vi "Main.vi"() -> ()   [LabVIEW 2017]
uses:
  Experiment States.ctl
  <vilib>/DAQmx/read.llb/DAQmx Read (Analog 1D DBL NChan 1Samp).vi
  <vilib>/DAQmx/miscellaneous.llb/DAQmx Fill In Error Info.vi
panel:
  in  "Lower Tower Delta P Channel":tag="cDAQ1Mod1/ai8"
  in  "Upper Tower Delta P Channel":tag="cDAQ1Mod1/ai8"
  out "Lower Tower Delta P":dbl(knob) scale=0.0..10.0
  out "Upper Tower Delta P":dbl(knob) scale=0.0..10.0
  in  "Maximum CO2 Concentration":dbl=20.0
  out "CO2 Concentration":cluster{"X":dbl, "Y":dbl}[](graph)
  in  "IR Sensor Channel":tag="cDAQ1Mod1/ai8"
  in  "End Experiment?":bool
  in  "Start":bool
  # "Set the above values before \nstarting the experiment"
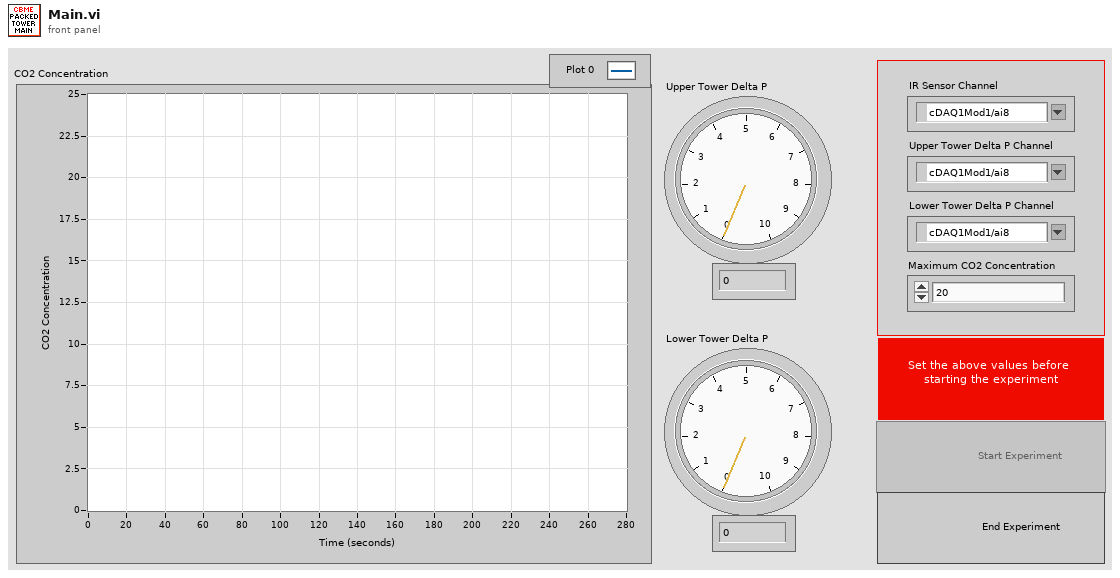
[diagram p1: front panel]
types:
  T1 = typedef "Experiment States.ctl" = enum16{"Setup", "Data Collection", "Export", "Finish"}
  T2 = enum8{"Enabled", "Disabled", "Disabled and Grayed Out"}
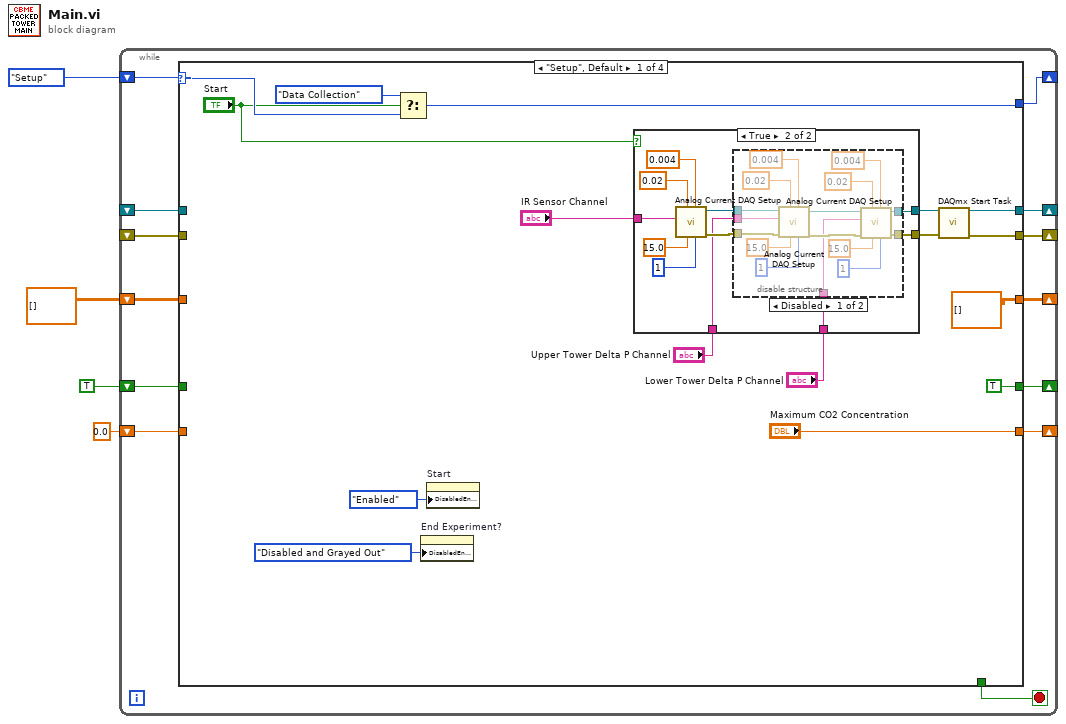
[diagram p0: block diagram]
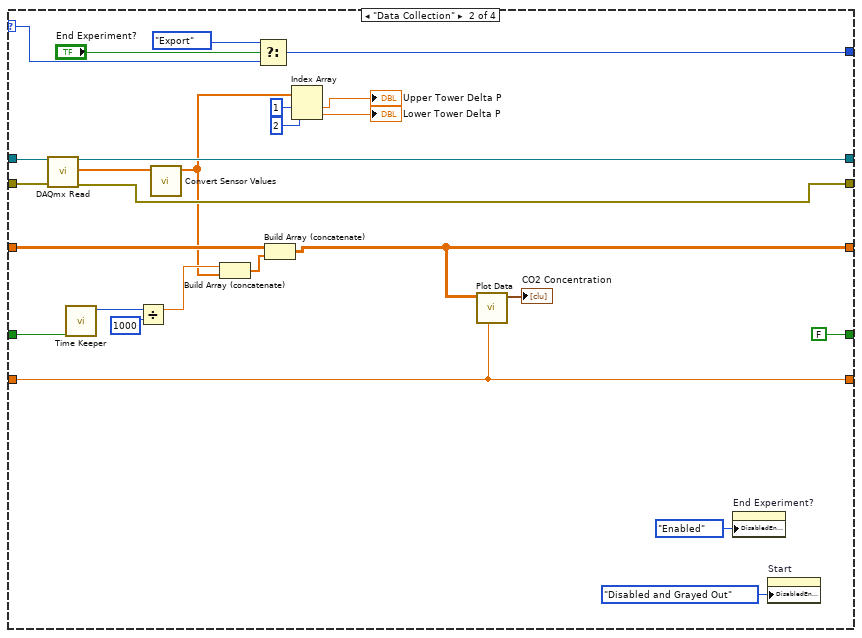
[diagram p4: hidden frame]
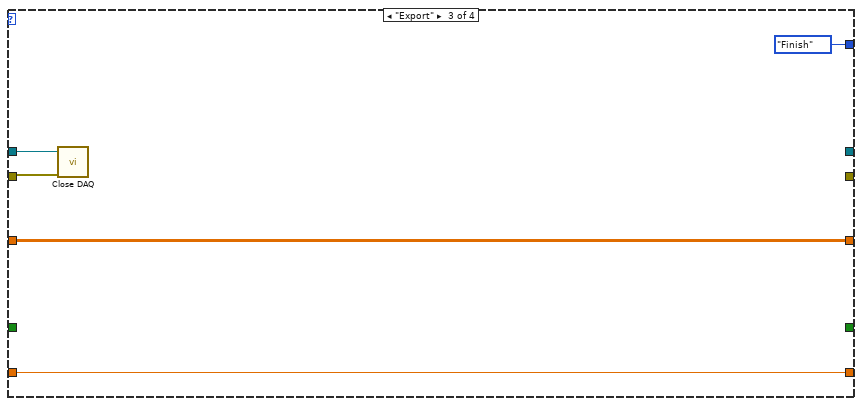
[diagram p5: hidden frame]
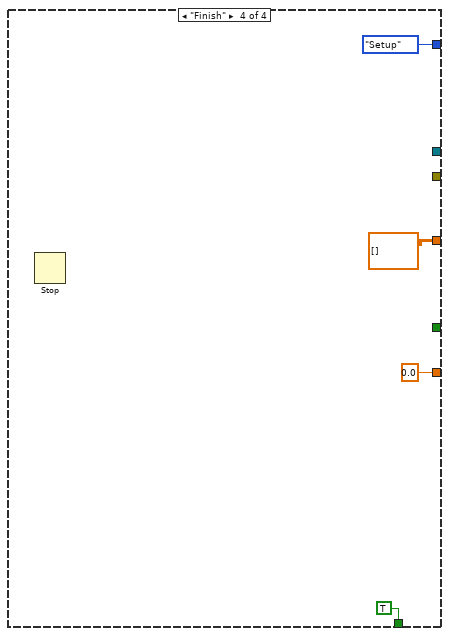
[diagram p6: hidden frame]
diagram:
  n1 = while {
    shift-right: [w16] -> _
    shift-left: Experiment_States."Setup" ("Enum") -> [w17]
    shift-right: [w13] -> _
    shift-left: _ -> [w11]
    shift-right: [w14] -> _
    shift-left: _ -> [w12]
    shift-right: [w5] -> _
    shift-left: TRUE ("Reset?") -> [w10]
    shift-right: [w8] -> _
    shift-left: dbl[][] [] -> [w9]
    shift-right: [w7] -> _
    shift-left: 0.0 ("IR Sensor Max Value") -> [w6]
    stop <- w15 stop-if-true
    n2 = case shown="\"Setup\", Default" w17 {
      selector: w17 -> [w33 w87 _ _]
      tunnel: [w31 w85 Experiment_States."Finish" ("Enum") Experiment_States."Setup" ("Enum")] -> w16
      tunnel: [_ _ _ TRUE] -> w15
      tunnel: [w27 w81 _ _] -> w14
      tunnel: [w26 w80 _ _] -> w13
      tunnel: w12 -> [_ w83 w92 _]
      tunnel: w11 -> [_ w82 w91 _]
      tunnel: w10 -> [_ w79 _ _]
      tunnel: w9 -> [_ w77 w90 _]
      tunnel: [dbl[][] [] w69 w90 dbl[][] []] -> w8
      tunnel: ["Maximum CO2 Concentration" w74 w89 0.0 ("IR Sensor Max Value")] -> w7
      tunnel: w6 -> [_ w74 w89 _]
      tunnel: [TRUE ("Reset?") FALSE ("Reset?") _ _] -> w5
      frame "Setup", Default {
        n3 = Select(t=Experiment_States."Data Collection", s="Start", f=w33) -> (s? t:f=w31:T1)
        n4 = property on="End Experiment?" class="Bool"("DisabledEnum"=T2."Disabled and Grayed Out" ("Disabled")) -> ()  [unwired: 2 in, 2 out]
        n5 = property on="Start" class="Bool"("DisabledEnum"=T2."Enabled" ("Disabled")) -> ()  [unwired: 2 in, 2 out]
        n6 = case shown="True" "Start" {
          tunnel: [_ w36] -> w29
          tunnel: [_ w35] -> w28
          tunnel: "IR Sensor Channel" -> [_ w42]
          tunnel: "Upper Tower Delta P Channel" -> [_ w37]
          tunnel: "Lower Tower Delta P Channel" -> [_ w34]
          frame False {
          }
          frame True {
            n7 = call "Analog Current DAQ Setup.vi"("samples per channel"=1, "minimum value"=0.004, "rate"=15.0 ("Sample Rate"), "maximum value"=0.02, "physical channels"=w42) -> ("error out"=w38:errorcluster, "task out"=w39:refnum<k21>)  [unwired: 5 in]
            n8 = disable-structure shown="Disabled" {
              disable-tunnel: w39 -> [w56 w62]
              disable-tunnel: w38 -> [w55 w61]
              disable-tunnel: w37 -> [w54 _]
              disable-tunnel: [w47 w62] -> w36
              disable-tunnel: [w46 w61] -> w35
              disable-tunnel: w34 -> [w45 _]
              frame Disabled {
                n9 = call "Analog Current DAQ Setup.vi"("samples per channel"=1, "minimum value"=0.004, "rate"=15.0 ("Sample Rate"), "maximum value"=0.02, "error in"=w55, "physical channels"=w54, "task in"=w56) -> ("error out"=w48:errorcluster, "task out"=w49:refnum<k21>)  [unwired: 3 in]
                n10 = call "Analog Current DAQ Setup.vi"("samples per channel"=1, "minimum value"=0.004, "rate"=15.0 ("Sample Rate"), "maximum value"=0.02, "error in"=w48, "physical channels"=w45, "task in"=w49) -> ("error out"=w46:errorcluster, "task out"=w47:refnum<k21>)  [unwired: 3 in]
              }
              frame Enabled {
              }
            }
          }
        }
        n11 = call <vilib>:"DAQmx Start Task.vi"("task/channels in"=w29, "error in"=w28) -> ("task out"=w27:refnum<k21>, "error out"=w26:errorcluster)  [unwired: 12 in]
      }
      frame "Data Collection" {
        n12 = call-poly <vilib>:"DAQmx Read.vi"("task/channels in"=w83, "error in"=w82) -> ("task out"=w81:refnum<k21>, "data"=w64:dbl[], "error out"=w80:errorcluster)  [unwired: 11 in]
        n13 = call "Time Keeper.vi"("Reset?"=w79) -> ("Time Elapsed (ms)"=w78:u32)  [unwired: 10 in]
        n14 = Divide(x=w78, y=u32 1000) -> (x/y=w71:dbl)
        n15 = call "Convert Sensor Values.vi"("ECE Units"=w64) -> ("CBME Units"=w63:dbl[])  [unwired: 10 in]
        n16 = Build Array (concatenate)(w71, w63) -> (w76:dbl[])
        n17 = Select(t=Experiment_States."Export", s="End Experiment?", f=w87) -> (s? t:f=w85:T1)
        n18 = Build Array (concatenate)(w77, w76) -> (w69:dbl[][])
        n19 = Index Array(array=w63, index #1=1 ("index"), index #2=2 ("index")) -> (element #1=→"Upper Tower Delta P":dbl, element #2=→"Lower Tower Delta P":dbl)
        n20 = call "Plot Data.vi"("Max Value"=w74, "Data"=w69) -> ("XY Graph"=→"CO2 Concentration":cluster{"X":dbl, "Y":dbl}[])  [unwired: 9 in]
        n21 = property on="End Experiment?" class="Bool"("DisabledEnum"=T2."Enabled" ("Disabled")) -> ()  [unwired: 2 in, 2 out]
        n22 = property on="Start" class="Bool"("DisabledEnum"=T2."Disabled and Grayed Out" ("Disabled")) -> ()  [unwired: 2 in, 2 out]
      }
      frame "Export" {
        n23 = call "Close DAQ.vi"("error in (no error)"=w91, "Refnum in"=w92) -> ()  [unwired: 10 in]
      }
      frame "Finish" {
        n24 = Stop() -> ()  [unwired: 1 in]
      }
    }
  }
